vi "Game Data Util.vi"   [LabVIEW 2025]
uses:
  Globals.vi
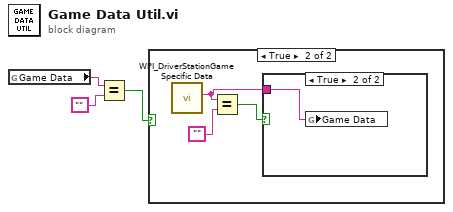
[diagram p0: block diagram]
diagram:
  n1 = global read "Globals.vi" "Game Data"() -> (w2:string)
  n2 = Equal?(x=w2, y="") -> (x = y?=w1:bool)
  n3 = case shown="True" w1 {
    frame False {
    }
    frame True {
      n4 = call <vilib>:"WPI_DriverStationGame Specific Data.vi"() -> ("Game Specific Data"=w4:string)  [unwired: 11 in]
      n5 = Equal?(x=w4, y="") -> (x = y?=w5:bool)
      n6 = case shown="True" w5 {
        tunnel: w4 -> [_ w7]
        frame False {
        }
        frame True {
          n7 = global write "Globals.vi" "Game Data"(w7) -> ()
        }
      }
    }
  }
